vi "Get Resource Name.vi"(8 "error in":errorcluster, 11 "FPGA Ref In":refnum<k20>) -> (0 "error out":errorcluster, 1 "alias":string, 2 "resource name":string, 3 "FPGA Ref Out":refnum<k20>)   [LabVIEW 2025, in "I2C Bus Monitor.lvclass"]
uses:
  <vilib>/nisyscfg/Filter Mode.ctl
  I2C Bus Monitor.lvclass
  I2C Bus Monitor.lvclass/I2C Bus Monitor.ctl
  <vilib>/nisyscfg/Close (Filter).vi
  <instrlib>/FlexRIO/API/Host/v1/NI FlexRIO/API/Get Property Reference - Fpga Small.vi
  <resource>/objmgr/nicriosae.rc
  <resource>/objmgr/niflexrioatomicsae.rc
  <vilib>/nisyscfg/nisyscfg.lvlib
  <resource>/objmgr/niflexrioapi.rc
  <instrlib>/FlexRIO/API/Host/v1/NI FlexRIO API v1.lvlib
  <vilib>/nisyscfg/Close (Resources).vi
  <vilib>/nisyscfg/Close (System).vi
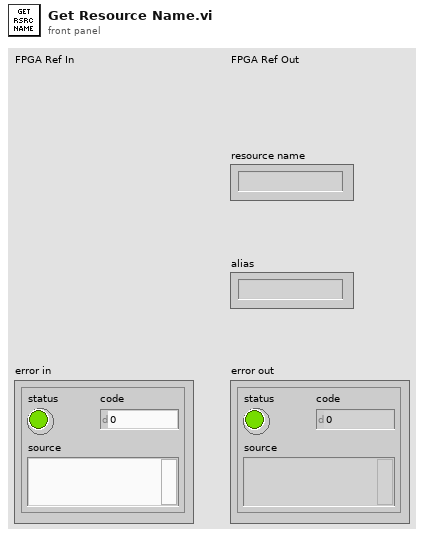
[diagram p1: front panel]
types:
  T1 = typedef "nisyscfg.lvlib/Filter Mode.ctl" = i32
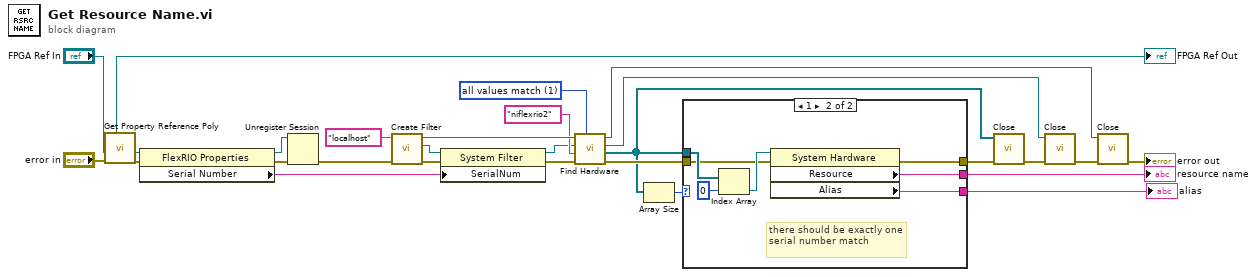
[diagram p0: block diagram]
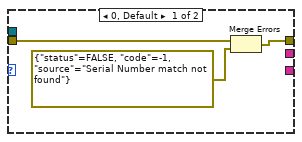
[diagram p2: hidden frame]
diagram:
  w27 = T1 1 items=["all values match"=1, "any value matches"=2, "values do not match"=3, "all properties exist"=4] ("filter mode (all values match)")
  n1 = call-poly <instrlib>:"Get Property Reference Poly.vi"("error in (no error)"="error in", "fpga interface in"="FPGA Ref In") -> ("error out"=w23:errorcluster, "property reference"=w24:refnum<k20>, "fpga interface out"=→"FPGA Ref Out":refnum<k20>)  [unwired: 4 in]
  n2 = property class="FlexRIO Properties"(reference=w24, error in=w23) -> (reference out=w7:refnum<k20>, error out=w9:errorcluster, "Serial Number"=w17:string)
  n3 = Unregister Session(8:w9, 11:w7) -> (0:w8:errorcluster)
  n4 = call <vilib>:"Create Filter.vi"("error in (no error)"=w8, "Session in"="localhost") -> ("error out"=w18:errorcluster, "Filter out"=w19:refnum<k20>, "Session out"=w28:refnum<k21>)  [unwired: 7 in]
  n5 = property class="System Filter"(reference=w19, error in=w18, "SerialNum"=w17) -> (reference out=w16:refnum<k20>, error out=w15:errorcluster)
  n6 = call <vilib>:"Find Hardware.vi"("Filter Mode (all values match)"=w27, "error in (no error)"=w15, "Experts"="niflexrio2", "Filter in"=w16, "Session in"=w28) -> ("error out"=w14:errorcluster, "Resources out"=w4:refnum<k20>[], "Filter out"=w26:refnum<k20>, "Session out"=w3:refnum<k21>)  [unwired: 3 out]
  n7 = Array Size(array=w4) -> (size(s)=w13:i32)
  n8 = case shown="1" w13 {
    tunnel: w14 -> [w30 w35]
    tunnel: [w31 w34] -> w5
    tunnel: w4 -> [_ w38]
    tunnel: [_ w33] -> w12
    tunnel: [_ w32] -> w11
    frame 0, Default {
      n9 = Merge Errors(w30, errorcluster {"status"=FALSE, "code"=-1, "source"="Serial Number match not found"} ("error constant")) -> (w31:errorcluster)
    }
    frame 1 {
      # "there should be exactly one serial number match"
      n10 = Index Array(array=w38, index=0) -> (element=w36:refnum<k20>)
      n11 = property class="System Hardware"(reference=w36, error in=w35) -> (error out=w34:errorcluster, "Resource"=w33:string, "Alias"=w32:string)  [unwired: 1 out]
    }
  }
  "resource name" <- w12
  "alias" <- w11
  n12 = call-poly <vilib>:"Close.vi"("error in (no error)"=w5, "Resources in"=w4) -> ("error out"=w2:errorcluster)  [unwired: 9 in]
  n13 = call-poly <vilib>:"Close.vi"("error in (no error)"=w2, "Filter in"=w26) -> ("error out"=w6:errorcluster)  [unwired: 9 in]
  n14 = call-poly <vilib>:"Close.vi"("error in (no error)"=w6, "Session in"=w3) -> ("error out"=→"error out":errorcluster)  [unwired: 9 in]
